vi "Get Variant.vi"(8 "error in (no error)":errorcluster, 11 "int32 in":refnum<class "sfixed32.lvclass">) -> (0 "error out":errorcluster, 2 "Variant":variant, 3 "int32 out":refnum<class "sfixed32.lvclass">)   [LabVIEW 2020, in "Protobuf RAW.lvlib" / "sfixed32.lvclass"]
uses:
  sfixed32.lvclass
  sfixed32.lvclass/sfixed32.ctl
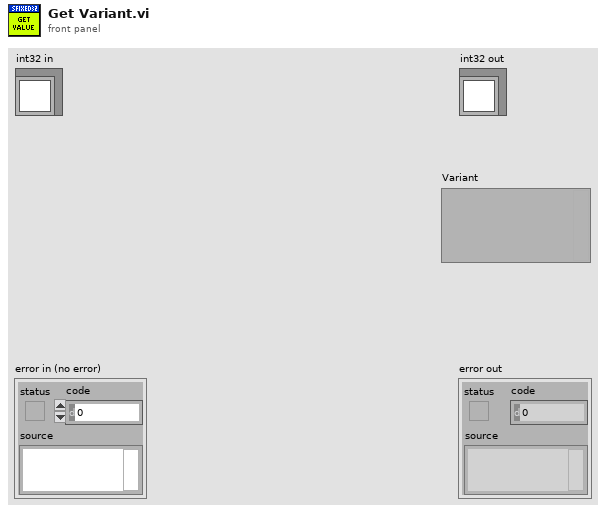
[diagram p1: front panel]
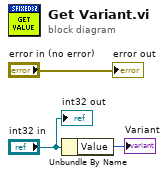
[diagram p0: block diagram]
diagram:
  n1 = Unbundle By Name("int32 in") -> ("Value"=→"Variant":i32)
  "error out" <- "error in (no error)"
  "int32 out" <- "int32 in"
